vi "CameraGetData.vi"(8 "error in (no error)":errorcluster, 10 "keep open?":bool, 11 "NIvision in":refnum<class "IMAQdx_Flea3_Firewire.lvclass">) -> (0 "error out":errorcluster, 2 "image_data":u16[][][](array[numeric]), 3 "NIvision out":refnum<class "IMAQdx_Flea3_Firewire.lvclass">)   [LabVIEW 2012, in "IMAQdx_Flea3_Firewire.lvclass"]
uses:
  <userlib>/bias2/classes/IMAQdx_Flea3_Firewire/IMAQdx_Flea3_Firewire.lvclass
  <userlib>/bias2/classes/IMAQdx_Flea3_Firewire/IMAQdx_Flea3_Firewire.lvclass/IMAQdx_Flea3_Firewire.ctl
  <vilib>/vision/driver/IMAQdx.llb/IMAQdx Buffer Number Mode.ctl
  <vilib>/vision/driver/NI_Vision_Acquisition_Software.lvlib
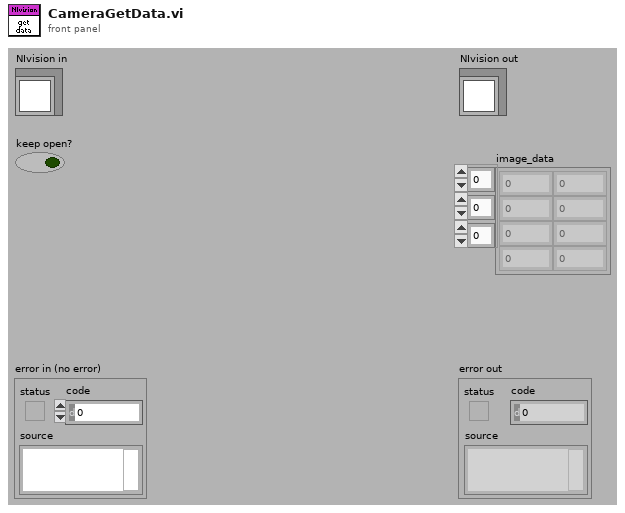
[diagram p1: front panel]
types:
  T1 = typedef "NI_Vision_Acquisition_Software.lvlib/IMAQdx Buffer Number Mode.ctl" = enum32{"Next", "Last", "Buffer Number"}
  T2 = typedef "IMAQ Image.ctl" = refnum<image>
  T3 = typedef "IMAQdx.ctl" = refnum<k21>
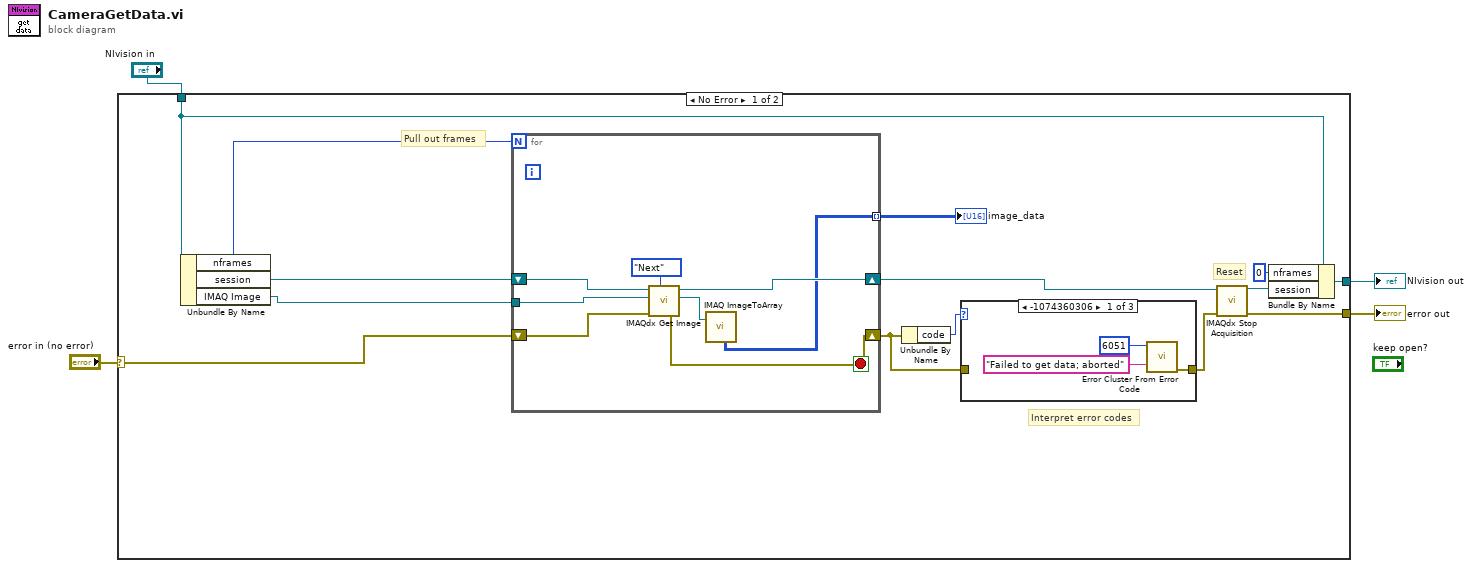
[diagram p0: block diagram]
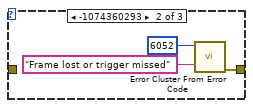
[diagram p2: hidden frame]
diagram:
  n1 = case shown="No Error" "error in (no error)" {
    selector: "error in (no error)" -> [w6 w34]
    tunnel: "NIvision in" -> [w17 w35]
    tunnel: [w10 w35] -> w2
    tunnel: [w8 w34] -> w1
    frame No Error {
      # "Interpret error codes"
      # "Reset"
      # "Pull out frames"
      n2 = Unbundle By Name(w17) -> ("nframes"=w16:i32, "session"=w7:refnum<k21>, "IMAQ Image"=w5:T2)
      n3 = for {
        N: w16 -> [_]
        tunnel: [w29] -> w11 mode=indexing
        shift-right: [w32] -> w18
        shift-left: w7 -> [w33]
        shift-right: [w28] -> w13
        shift-left: w6 -> [w31]
        tunnel: w5 -> [w27]
        stop <- w28 stop-if-true
        n4 = call <vilib>:"IMAQdx Get Image.vi"("Buffer Number Mode (Next)"=IMAQdx_Buffer_Number_Mode."Next", "error in"=w31, "Image In"=w27, "Session In"=w33) -> ("error out"=w28:errorcluster, "Image Out"=w26:T2, "Session Out"=w32:T3)  [unwired: 4 in, 1 out]
        n5 = call "IMAQ ImageToArray"("Image"=w26) -> ("Image Pixels (U16)"=w29:u16[][])  [unwired: 2 in, 5 out]
      }
      "image_data" <- w11
      n6 = Unbundle By Name(w13) -> ("code"=w14:i32)
      n7 = case shown="-1074360306" w14 {
        tunnel: [w19 w22 w25] -> w12
        tunnel: w13 -> [_ _ w25]
        frame -1074360306 {
          n8 = call <vilib>:"Error Cluster From Error Code.vi"("error message (\"\")"="Failed to get data; aborted" ("error message (\"\")"), "error code (0)"=6051) -> ("error out"=w19:errorcluster)  [unwired: 7 in]
        }
        frame -1074360293 {
          n9 = call <vilib>:"Error Cluster From Error Code.vi"("error message (\"\")"="Frame lost or trigger missed" ("error message (\"\")"), "error code (0)"=6052) -> ("error out"=w22:errorcluster)  [unwired: 7 in]
        }
        frame Default {
        }
      }
      n10 = call <vilib>:"IMAQdx Stop Acquisition.vi"("error in"=w12, "Session In"=w18) -> ("error out"=w8:errorcluster, "Session Out"=w9:T3)  [unwired: 8 in]
      n11 = Bundle By Name(cluster=w17, "nframes"=0, "session"=w9) -> (w10:refnum<class "IMAQdx_Flea3_Firewire.lvclass">)
    }
    frame Error {
    }
  }
  "NIvision out" <- w2
  "error out" <- w1
